vi "HFRR ADV v012 new software.vi"() -> ()   [LabVIEW 2025] (continued)
                n3074 = local read "Ref A Test Date :"() -> (→"TITTLE 4":string)
                n3075 = local read "Temperature before test 3"() -> (w3788:dbl)
                n3076 = local read "Temperature before test 3"() -> (→"Temperature after test 5":dbl)
                n3077 = local read "Temperature after test 3"() -> (→"Temperature after test 4":dbl)
                n3078 = local read "Humidity before test 3"() -> (→"Humidity before test 4":dbl)
                n3079 = local write "Temperature before test 3"(w3788) -> ()
                n3080 = local read "image data"() -> (w3779:T15)
                n3081 = String To Path(string="C:\\LAB-IQ\\im\\Temp_resized.jpg") -> (path=w3780:path)
                "path 2" <- w3780
                n3082 = call <vilib>:"Write JPEG File.vi"("image data"=w3779, "path to JPEG file"=w3780) -> ()  [unwired: 8 in, 2 out]
                "Ref A Test Date :" <- "Ref A Test Date :"
                "Ref B Test Date :" <- "Ref B Test Date :"
                "Ref B Scar Value :" <- "Ref B Scar Value :"
                "Ref A Scar Value :" <- "Ref A Scar Value :"
              }
              frame #1 {
                (unwired) HTML_Report_Image_Alignment."MIDDLE" ("alignment (default)")
                w3816 = u16 0 items=["portrait", "landscape"] ("orientation (portrait)")
                (unwired) HTML_Report_Image_Alignment."ABSMIDDLE" ("alignment (default)")
                (unwired) "TESTED BY : "
                (unwired) "TESTED DATE :"
                (unwired) "SAMPLE ID : "
                (unwired) "SAMPLE DESIGN : "
                w3849 = "\r"
                # "add image"
                n3083 = Wait (ms)(milliseconds to wait=u32 20) -> ()  [unwired: 1 out]
                n3084 = local read "Sample ID  2"() -> (w3842:string)
                n3085 = local read "Wear Scar X"() -> (w3814:dbl)
                "Length ( microns ) 2" <- w3814
                n3086 = local read "Wear Scar Y"() -> (w3813:dbl)
                "Wear Scar Y ( microns ) :" <- w3813
                n3087 = local read "Test Date 2"() -> (w3843:string)
                n3088 = local read "Tested by 2"() -> (w3844:string)
                n3089 = local read "String 46"() -> (w3840:string)
                n3090 = local read "String 48"() -> (w3846:string)
                n3091 = local read "String 47"() -> (w3845:string)
                n3092 = local read "String 49"() -> (w3847:string)
                n3093 = local read "String 10"() -> (w3800:string)
                n3094 = local read "s.NO 2"() -> (w3841:string)
                n3095 = Add(x=w3814, y=w3813) -> (x+y=w3812:dbl)
                n3096 = call <vilib>:"New Report.vi"("report type"=enum16{"Standard Report", "HTML"}."HTML") -> ("report out"=w3820:refnum<class "NI_report.lvclass">, "error out"=w3818:errorcluster)  [unwired: 13 in]
                n3097 = Concatenate Strings(w3849, w3840, w3841, w3849, w3846, w3842, w3849, w3845, w3843, w3849, w3847, w3844, w3849) -> (→"test by 2":string)
                n3098 = Concatenate Strings("C:\\LAB-IQ\\Data\\" ("string"), w3800, ".jpg" ("string")) -> ()  [unwired: 1 out]
                n3099 = Divide(x=w3812, y=2.0) -> (x/y=→"Mean Wear ( microns) :":dbl)
                n3100 = call-dynamic "Set Report Orientation.vi"("report in"=w3820, "orientation (portrait)"=w3816, "error in (no error)"=w3818) -> ("report out"=w3819:refnum<class "NI_report.lvclass">, "error out"=w3817:errorcluster)  [unwired: 11 in]
                n3101 = for {
                  N: 5 -> [_]
                  tunnel: w3819 -> [w3870]
                  tunnel: [w3869] -> w3798
                  tunnel: w3817 -> [w3868]
                  tunnel: [w3867] -> w3797
                  n3102 = call-dynamic "Set Report Tab Width.vi"("report in"=w3870, "error in (no error)"=w3868) -> ("report out"=w3869:refnum<class "NI_report.lvclass">, "error out"=w3867:errorcluster)  [unwired: 12 in]
                }
                n3103 = local read "TITTLE"() -> (w3815:string)
                n3104 = call-dynamic "Set Report Header Text.vi"("report in"=w3798, "center header text"=w3815, "error in (no error)"=w3797) -> ("report out"=w3836:refnum<class "NI_report.lvclass">, "error out"=w3835:errorcluster)  [unwired: 11 in]
                n3105 = for {
                  N: 1 -> [_]
                  tunnel: [w3874] -> w3822
                  tunnel: [w3873] -> w3821
                  tunnel: w3836 -> [w3872]
                  tunnel: w3835 -> [w3871]
                  n3106 = call-dynamic "New Report Line.vi"("report in"=w3872, "error in (no error)"=w3871) -> ("report out"=w3874:refnum<class "NI_report.lvclass">, "error out"=w3873:errorcluster)  [unwired: 12 in]
                }
                n3107 = for {
                  N: 2 -> [_]
                  tunnel: [w3866] -> w3828
                  tunnel: [w3865] -> w3827
                  tunnel: w3822 -> [w3864]
                  tunnel: w3821 -> [w3863]
                  n3108 = call-dynamic "New Report Line.vi"("report in"=w3864, "error in (no error)"=w3863) -> ("report out"=w3866:refnum<class "NI_report.lvclass">, "error out"=w3865:errorcluster)  [unwired: 12 in]
                }
                n3109 = for {
                  N: 25 -> [_]
                  tunnel: w3828 -> [w3862]
                  tunnel: w3827 -> [w3860]
                  tunnel: [w3861] -> w3831
                  tunnel: [w3859] -> w3830
                  n3110 = call-dynamic "Set Report Tab Width.vi"("report in"=w3862, "error in (no error)"=w3860) -> ("report out"=w3861:refnum<class "NI_report.lvclass">, "error out"=w3859:errorcluster)  [unwired: 12 in]
                }
                n3111 = control-ref of="Tab Control 9"() -> (w3826:refnum<vi>)
                n3112 = call-dynamic "Append Control Image to Report.vi"("report in"=w3831, "alignment (default)"=HTML_Report_Image_Alignment."ABSMIDDLE", "ctrl reference"=w3826, "error in (no error)"=w3830) -> ("report out"=w3825:refnum<class "NI_report.lvclass">, "error out"=w3824:errorcluster)  [unwired: 8 in, 2 out]
                n3113 = for {
                  N: 3 -> [_]
                  tunnel: [w3858] -> w3809
                  tunnel: [w3857] -> w3808
                  tunnel: w3825 -> [w3856]
                  tunnel: w3824 -> [w3855]
                  n3114 = call-dynamic "New Report Line.vi"("report in"=w3856, "error in (no error)"=w3855) -> ("report out"=w3858:refnum<class "NI_report.lvclass">, "error out"=w3857:errorcluster)  [unwired: 12 in]
                }
                n3115 = for {
                  N: 100 -> [_]
                  tunnel: w3809 -> [w3854]
                  tunnel: w3808 -> [w3852]
                  tunnel: [w3853] -> w3805
                  tunnel: [w3851] -> w3803
                  n3116 = call-dynamic "Set Report Tab Width.vi"("report in"=w3854, "error in (no error)"=w3852) -> ("report out"=w3853:refnum<class "NI_report.lvclass">, "error out"=w3851:errorcluster)  [unwired: 12 in]
                }
                n3117 = String To Path(string="C:\\LAB-IQ\\im\\Temp_resized.jpg") -> (path=w3795:path)
                n3118 = call-poly <vilib>:"Append Image to Report.vi"("report in"=w3805, "path or URL of image"=w3795, "error in (no error)"=w3803) -> ("report out"=w3804:refnum<class "NI_report.lvclass">, "error out"=w3802:errorcluster)  [unwired: 9 in, 2 out]
                n3119 = call-poly <vilib>:"Open HTML Report in Browser.vi"("report in"=w3804, "error in (no error)"=w3802) -> ("report out"=w3839:refnum<class "NI_report.lvclass">, "error out"=w3838:errorcluster)  [unwired: 11 in, 1 out]
                n3120 = call-dynamic "Dispose Report.vi"("report in"=w3839, "error in (no error)"=w3838) -> ()  [unwired: 13 in, 1 out]
              }
              frame #2 {
              }
              frame #3 {
                n3121 = disable-structure shown="Disabled" {
                  frame Disabled {
                    n3122 = local read "String 10"() -> (w3879:string)
                    n3123 = Concatenate Strings("C:\\LAB-IQ-NXT\\Data\\" ("string"), w3879, ".jpg" ("string")) -> (w3877:string)
                    n3124 = String To Path(string=w3877) -> (path=w3876:path)
                    n3125 = Delete(path (use dialog)=w3876) -> ()  [unwired: 4 in, 3 out]
                  }
                  frame Enabled {
                  }
                }
                n3126 = local write "Print 2"(FALSE ("Print")) -> ()
              }
            }
          }
        }
      }
    }
    n3127 = property on="SetTemp" class="DigNum (strict)"("Disabled"=w1815) -> ()  [unwired: 2 in, 2 out]
    n3128 = Multiply(x=w1805, y=w1807) -> (x*y=w1806:dbl)
    n3129 = local read "MWSD"() -> (w1804:dbl)
    n3130 = Add(x=w1806, y=w1804) -> (x+y=→"WS1.4":dbl)
    n3131 = Wait (ms)(milliseconds to wait=u32 50) -> ()  [unwired: 1 out]
    n3132 = Wait (ms)(milliseconds to wait=u32 50) -> ()  [unwired: 1 out]
    n3133 = local read "Quit"() -> (w1803:bool)
  }
  n3134 = VISA Close(VISA resource name=w52, error in (no error)=w51) -> (error out=w49:errorcluster)
  n3135 = call <vilib>:"Clear Errors.vi"("error in (no error)"=w49) -> ()  [unwired: 5 in, 2 out]
  n3136 = VISA Close(VISA resource name=w37, error in (no error)=w36) -> ()  [unwired: 1 out]
  n3137 = while {
    tunnel: [w4040] -> w46
    shift-right: [w4033] -> _
    shift-left: 0.0 -> [w4036]
    shift-right: [w4032] -> _
    shift-left: 0.0 -> [w4035]
    shift-right: [w4031] -> _
    shift-left: 400.0 ("vc_cmd") -> [w4034]
    stop <- w4040 stop-if-true
    # "PID LOGIC"
    n3138 = local read "RUN"() -> (w4038:bool)
    n3139 = local read "Auto Start Temp"() -> (w4027:bool)
    n3140 = local read "Auto Start Test"() -> (w4037:bool)
    n3141 = local read "START TEMP"() -> (w4029:bool)
    n3142 = And(x=w4027, y=w4037) -> (x .and. y?=w4028:bool)
    n3143 = Or(x=w4038, y=w4028) -> (x .or. y?=w4039:bool)
    n3144 = And(x=w4039, y=w4029) -> (x .and. y?=w4030:bool)
    n3145 = Wait (ms)(milliseconds to wait=u32 20) -> ()  [unwired: 1 out]
    n3146 = case shown="True" w4030 {
      tunnel: [400.0 ("out_vc_cmd") w4060] -> w4031
      tunnel: [w4043 w4062] -> w4032
      tunnel: [w4043 w4061] -> w4033
      tunnel: w4036 -> [_ w4051]
      tunnel: w4035 -> [_ w4050]
      tunnel: w4034 -> [_ w4049]
      frame False {
        w4043 = 0.0 ("error_out")
      }
      frame True {
        n3147 = local read "Set Strk"() -> (w4046:dbl)
        n3148 = local read "LVDT STROKE"() -> (w4044:dbl)
        n3149 = Add(x=w4046, y="Add up Stroke") -> (x+y=w4047:dbl)
        n3150 = formula code="// Zero-Hardcode Explicit Positional-Form PID Engine\n// Inputs: target_stroke, measured_stroke, dt, prev_error, integral_accumulator_in, prev_vc_cmd\n//         kp, ki, kd, max_step_change, max_amplitude, min_amplitude, startup_cmd\n// Outputs: vc_cmd, error_out, out_error, integral_accumulator_out, out_vc_cmd\n\n// 1. Calculate Tracking Error\nfloat current_error = target_stroke - measured_stroke;\nerror_out = current_error;\n\n// 2. Compute Proportional Term\nfloat p_term = kp * current_error;\n\n// 3. Compute Derivative Term\nfloat d_term = 0.0;\nif (dt > 0.0) {\n    d_term = kd * ((current_error - prev_error) / dt);\n}\n\n// 4. Update and Accumulate Integral Term\nfloat current_integral = integral_accumulator_in + (current_error * dt);\nfloat i_term = ki * current_integral;\n\n// 5. Calculate Ideal Target Command\nfloat ideal_command = startup_cmd + p_term + i_term + d_term;\n\n// 6. Anti-Windup Protection (Back-calculation method)\nif (ideal_command > max_amplitude) {\n    float excess = ideal_command - max_amplitude;\n    if (ki > 0.0) {\n        current_integral -= excess / ki;\n    }\n    ideal_command = max_amplitude;\n} else if (ideal_command < min_amplitude) {\n    float excess = ideal_command - min_amplitude;\n    if (ki > 0.0) {\n        current_integral -= excess / ki;\n    }\n    ideal_command = min_amplitude;\n}\n\n// 7. Apply Loop Rate Limiting (Protects voice coil from large voltage steps)\nfloat raw_adjustment = ideal_command - prev_vc_cmd;\n\nif (raw_adjustment > max_step_change) {\n    raw_adjustment = max_step_change;\n} else if (raw_adjustment < -max_step_change) {\n    raw_adjustment = -max_step_change;\n}\n\nfloat next_vc_cmd = prev_vc_cmd + raw_adjustment;\n\n// Final Output Safety Safeguard Clamping\nif (next_vc_cmd > max_amplitude) {\n    next_vc_cmd = max_amplitude;\n} else if (next_vc_cmd < min_amplitude) {\n    next_vc_cmd = min_amplitude;\n}\n\n// 8. Map to Shift Registers for memory persistence\nvc_cmd = next_vc_cmd;\nout_error = current_error;                     \nintegral_accumulator_out = current_integral;  \nout_vc_cmd = next_vc_cmd;"("target_stroke"=w4047, "measured_stroke"=w4044, "dt"="dt", "integral_accumulator_in"=w4050, "prev_error"=w4051, "prev_vc_cmd"=w4049, "kp"="kp", "ki"="ki", "kd"="kd", "max_step_change"="max_step_change", "max_amplitude"="max_amplitude", "min_amplitude"="min_amplitude", "startup_cmd"="startup_cmd") -> ("vc_cmd"=w4066:dbl, "out_error"=w4061:dbl, "integral_accumulator_out"=w4062:dbl, "out_vc_cmd"=w4060:dbl)  [unwired: 1 out]
        "output Vpp" <- w4066
        n3151 = Number To Fractional String(number=w4066, precision (6)=i16 1) -> (F-format string=w4064:string)  [unwired: 2 in]
        n3152 = Concatenate Strings("DAC;" ("string"), w4064) -> (w4048:string)
        n3153 = local write "Command"(w4048) -> ()
        "prev_error" <- w4051
        "integral_accumulator_in" <- w4050
        "prev_vc_cmd" <- w4049
      }
    }
    n3154 = local read "Quit"() -> (w4040:bool)
  }
  n3155 = Or(x=w42, y=w41) -> (x .or. y?=w43:bool)
  n3156 = Or(x=w39, y=w43) -> (x .or. y?=w48:bool)
  n3157 = control-ref of="new picture"() -> ()  [unwired: 1 out]
  n3158 = Or(x=w54, y=w48) -> (x .or. y?=w45:bool)
  n3159 = Or(x=w45, y=w46) -> (x .or. y?=w40:bool)
  n3160 = while {
    tunnel: [w4067] -> w53
    i -> [w4074]
    stop <- w4067 stop-if-true
    n3161 = local read "Quit"() -> (w4067:bool)
    n3162 = Equal To 0?(x=w4074) -> (x = 0?=w4072:bool)
    n3163 = call "Elapsed Time3"("Time Target (s)"=45.0, "Auto Reset"=TRUE) -> ("Time has Elapsed"=w4071:bool)  [unwired: 10 in, 7 out]
    n3164 = Wait (ms)(milliseconds to wait=u32 50) -> ()  [unwired: 1 out]
    n3165 = Or(x=w4071, y=w4072) -> (x .or. y?=w4073:bool)
    n3166 = case shown="True" w4073 {
      frame False {
      }
      frame True {
        n3167 = call <vilib>:"System Exec.vi"("run minimized? (F)"=TRUE, "error in (no error)"="error in (no error)", "command line"="powercfg.exe -change -monitor-timeout-ac 0") -> ("error out"=w4085:errorcluster)  [unwired: 5 in, 3 out]
        n3168 = call <vilib>:"System Exec.vi"("run minimized? (F)"=TRUE, "error in (no error)"=w4085, "command line"="powercfg.exe -change -disk-timeout-ac 0") -> ("error out"=w4084:errorcluster)  [unwired: 5 in, 3 out]
        n3169 = call <vilib>:"System Exec.vi"("run minimized? (F)"=TRUE, "error in (no error)"=w4084, "command line"="powercfg.exe -change -standby-timeout-ac 0") -> ("error out"=w4083:errorcluster)  [unwired: 5 in, 3 out]
        n3170 = call <vilib>:"System Exec.vi"("run minimized? (F)"=TRUE, "error in (no error)"=w4083, "command line"="powercfg.exe -change -hibernate-timeout-ac 0") -> ("error out"=w4082:errorcluster)  [unwired: 5 in, 3 out]
        n3171 = call <vilib>:"Simple Error Handler.vi"("error in (no error)"=w4082) -> ("error out"=w4088:errorcluster)  [unwired: 4 in, 4 out]
        n3172 = call <vilib>:"Clear Errors.vi"("error in (no error)"=w4088) -> ("error out"=→"error out":errorcluster)  [unwired: 5 in, 1 out]
      }
    }
  }
  n3173 = Compound Arithmetic op=OR(w56, w40, w53) -> (w55:bool)
  n3174 = flat-sequence {
    tunnel: w55 -> [_]
    tunnel: [w4090] -> w18
    tunnel: w18 -> [_]
    frame #0 {
      n3175 = call "CLOSE CONNECTION.vi"() -> ("error out"=w4090:errorcluster)  [unwired: 11 in]
    }
    frame #1 {
      n3176 = Quit LabVIEW(quit? (T)=TRUE) -> ()
      n3177 = local write "Quit"(FALSE ("EXIT")) -> ()
    }
  }
  n3178 = property on="Heater Button" class="Bool (strict)"("Visible"=TRUE) -> ()  [unwired: 2 in, 2 out]
  n3179 = disable-structure shown="Disabled" {
    disable-tunnel: _ -> [w4096 _]
    disable-tunnel: _ -> [w4093 _]
    disable-tunnel: _ -> [w4094 _]
    frame Disabled {
      n3180 = disable-structure shown="Disabled" {
        disable-tunnel: [w4103 _] -> w4095
        frame Disabled {
          n3181 = while {
            shift-right: [w4145] -> w4101
            shift-left: errorcluster {"status"=TRUE, "code"=0, "source"="Init"} ("error out") -> [w4110]
            shift-right: [w4144] -> w4100
            shift-left: _ -> [w4111]
            shift-right: [w4143] -> _
            shift-left: "" -> [w4142]
            tunnel: [w4104] -> w4103
            shift-right: ["Set Rh"] -> _
            shift-left: 0.0 ("Set Rh") -> [w4136]
            tunnel: [w4113] -> _
            i -> [w4113]
            stop <- w4104 stop-if-true
            n3182 = flat-sequence {
              tunnel: w4110 -> [w4148]
              tunnel: [w4148] -> w4109
              frame #0 {
                n3183 = Wait (ms)(milliseconds to wait=u32 200) -> ()  [unwired: 1 out]
              }
            }
            n3184 = local read "Com Port 3"() -> (w4112:refnum<visa-resource-name>)
            n3185 = local read "Humidity Str Rec"() -> (w4114:string)
            n3186 = Not Equal?(x="Set Rh", y=w4136) -> (x != y?=w4141:bool)
            n3187 = Number To Decimal String(number="Set Rh") -> (decimal integer string=w4139:string)  [unwired: 1 in]
            n3188 = Not Equal?(x=w4112, y=w4111) -> (x != y?=w4107:bool)
            n3189 = Concatenate Strings("#setPoint00" ("string"), w4139) -> (w4140:string)
            n3190 = case shown="False" w4141 {
              tunnel: w4140 -> [_ w4160]
              frame False {
                n3191 = local read "Humidity"() -> (w4157:bool)
                n3192 = case shown="True" w4157 {
                  frame False {
                    n3193 = local write "Humidity Str Send"("stop" ("Humidity Str Send")) -> ()
                  }
                  frame True {
                    n3194 = local write "Humidity Str Send"("start" ("Humidity Str Send")) -> ()
                  }
                }
              }
              frame True {
                n3195 = local write "Humidity Str Send"(w4160) -> ()
              }
            }
            n3196 = Or(x=w4107) -> (y=w4105:bool, x .or. y?=w4106:bool)
            n3197 = String Subset(string=w4114, offset (0)=7) -> (substring=w4129:string)  [unwired: 1 in]
            n3198 = Match Pattern(string=w4114, regular expression="?") -> (offset past match=w4132:i32)  [unwired: 1 in, 3 out]
            n3199 = Match Pattern(string=w4114, regular expression="v") -> (offset past match=w4135:i32)  [unwired: 1 in, 3 out]
            n3200 = case shown="True" w4106 {
              tunnel: w4109 -> [w4146 _]
              tunnel: [w4146 errorcluster {"status"=TRUE, "code"=0, "source"="Init"} ("error out")] -> w4108
              frame False {
              }
              frame True {
              }
            }
            n3201 = Equal?(x=w4132, y=-1) -> (x = y?=w4116:bool)
            n3202 = Match Pattern(string=w4129, regular expression="g") -> (after substring=w4130:string, offset past match=w4121:i32)  [unwired: 1 in, 2 out]
            n3203 = Match Pattern(string=w4129, regular expression="y") -> (after substring=w4128:string, offset past match=w4122:i32)  [unwired: 1 in, 2 out]
            n3204 = Greater?(x=w4122, y=w4121) -> (0:w4127:bool)
            n3205 = Greater Or Equal To 0?(x=w4122) -> (x >= 0?=w4119:bool)
            n3206 = Greater Or Equal To 0?(x=w4121) -> (x >= 0?=w4120:bool)
            n3207 = Or(x=w4119, y=w4120) -> (x .or. y?=w4118:bool)
            n3208 = Greater Or Equal To 0?(x=w4135) -> (x >= 0?=w4117:bool)
            n3209 = Select(t=w4128, s=w4127, f=w4130) -> (s? t:f=w4123:string)
            n3210 = case shown="Error" w4108 {
              selector: w4108 -> [w4173 w4219]
              tunnel: [w4171 w4212] -> w4145
              tunnel: w4111 -> [w4174 w4218]
              tunnel: [w4172 w4221] -> w4144
              tunnel: w4142 -> [w4161 w4220]
              tunnel: [w4168 w4220] -> w4143
              frame No Error {
                n3211 = call "Elapsed Time7"() -> ("Time has Elapsed"=w4167:bool)  [unwired: 12 in, 7 out]
                n3212 = Not Equal?(x="Humidity Str Send", y=w4161) -> (x != y?=w4163:bool)
                n3213 = Or(x=w4163, y=w4167) -> (x .or. y?=w4166:bool)
                n3214 = Select(t="Humidity Str Send", s=w4163, f="vals" ("regular expression")) -> (s? t:f=w4162:string)
                n3215 = Or(x=w4166, y="Send") -> (x .or. y?=w4170:bool)
                n3216 = case shown="True" w4170 {
                  tunnel: [w4177 w4182] -> w4171
                  tunnel: w4174 -> [w4176 w4190]
                  tunnel: w4173 -> [w4177 w4189]
                  tunnel: [w4176 w4183] -> w4172
                  tunnel: w4162 -> [_ w4188]
                  tunnel: [w4175 w4179] -> w4168
                  tunnel: "Humidity Str Send" -> [_ w4180]
                  tunnel: w4163 -> [_ w4181]
                  tunnel: w4161 -> [w4175 w4178]
                  frame False {
                  }
                  frame True {
                    n3217 = flat-sequence {
                      tunnel: w4190 -> [w4198]
                      tunnel: w4189 -> [w4197]
                      tunnel: w4188 -> [w4194]
                      tunnel: [w4196] -> w4187
                      tunnel: [w4195] -> w4186
                      tunnel: w4187 -> [w4201]
                      tunnel: w4186 -> [w4200]
                      tunnel: [w4201] -> w4185
                      tunnel: [w4200] -> w4184
                      tunnel: w4185 -> [w4208]
                      tunnel: w4184 -> [w4207]
                      tunnel: [w4206] -> w4183
                      tunnel: [w4205] -> w4182
                      frame #0 {
                        n3218 = local write "Ser Led"(TRUE ("Boolean 4")) -> ()
                        n3219 = Concatenate Strings(w4194, "\r") -> (w4193:string)
                        n3220 = VISA Write(VISA resource name=w4198, write buffer=w4193, error in (no error)=w4197) -> (VISA resource name out=w4196:refnum<visa-resource-name>, error out=w4195:errorcluster)  [unwired: 1 out]
                      }
                      frame #1 {
                        n3221 = Wait (ms)(milliseconds to wait="wait") -> ()  [unwired: 1 out]
                      }
                      frame #2 {
                        w4203 = FALSE ("Send")
                        n3222 = property class="Instr"(reference=w4208, error in=w4207) -> (reference out=w4209:refnum<visa-resource-name>, error out=w4210:errorcluster, "Serial Settings:Number of Bytes at Serial Port"=w4202:u32)
                        n3223 = local write "Send"(w4203) -> ()
                        n3224 = local write "Ser Led"(w4203) -> ()
                        n3225 = VISA Read(VISA resource name=w4209, byte count=w4202, error in (no error)=w4210) -> (VISA resource name out=w4206:refnum<visa-resource-name>, read buffer=→"Humidity Str Rec":string, error out=w4205:errorcluster)  [unwired: 1 out]
                      }
                    }
                    n3226 = Select(t=w4180, s=w4181, f=w4178) -> (s? t:f=w4179:string)
                  }
                }
              }
              frame Error {
                w4226 = u16 0 items=["None"=0, "XON/XOFF"=1, "RTS/CTS"=2, "DTR/DSR"=4] ("flow control")
                w4222 = u16 0 items=["None", "Odd", "Even", "Mark", "Space"] ("parity")
                w4225 = u16 10 items=["1.0"=10, "1.5"=15, "2.0"=20] ("stop bits")
                n3227 = VISA Close(VISA resource name=w4218, error in (no error)=w4219) -> (error out=w4217:errorcluster)
                n3228 = local write "humid"("" ("humid")) -> ()
                n3229 = local write "Humidity Str Rec"("" ("Humidity Str Rec")) -> ()
                n3230 = call <vilib>:"Clear Errors.vi"("error in (no error)"=w4217) -> ("error out"=w4216:errorcluster)  [unwired: 5 in, 1 out]
                n3231 = local read "Com Port 3"() -> (w4215:refnum<visa-resource-name>)
                n3232 = call-poly "VISA Configure Serial Port"("VISA resource name"=w4215, "timeout (10sec)"=u32 1000, "termination char\n(0xA = '\\n' = LF)"=u8 10 ("termination char\n(0xA = '\\n' = LF)"), "Enable Termination\nChar (T)"=FALSE ("Enable Termination Char (T)"), "data bits (8)"=u16 8 ("data bits"), "parity (0:none)"=w4222, "error in (no error)"=w4216, "stop bits (10: 1 bit)"=w4225, "flow control (0:none)"=w4226) -> ("VISA resource name out"=w4221:refnum<visa-resource-name>, "baud rate (9600)"=w4213:u32, "error out"=w4212:errorcluster)  [unwired: 4 in]
              }
            }
            n3233 = Compound Arithmetic op=AND(w4117, w4116, w4118) -> (w4115:bool)
            n3234 = case shown="True" w4115 {
              tunnel: w4114 -> [_ _]
              tunnel: w4123 -> [_ w4153]
              frame False {
              }
              frame True {
                w4151 = " " ("regular expression")
                n3235 = Match Pattern(string=w4153, regular expression=" ") -> (after substring=w4155:string)  [unwired: 1 in, 3 out]
                n3236 = Match Pattern(string=w4155, regular expression=w4151) -> (before substring=→"humid":string, after substring=w4152:string)  [unwired: 1 in, 2 out]
                n3237 = Match Pattern(string=w4152, regular expression=w4151) -> (before substring=→"temp_@Rh sensor":string)  [unwired: 1 in, 3 out]
              }
            }
            n3238 = local read "Quit"() -> (w4104:bool)
          }
          n3239 = VISA Close(VISA resource name=w4100, error in (no error)=w4101) -> (error out=w4097:errorcluster)
          n3240 = call <vilib>:"Clear Errors.vi"("error in (no error)"=w4097) -> ()  [unwired: 5 in, 2 out]
        }
        frame Enabled {
        }
      }
    }
    frame Enabled {
    }
  }
  n3241 = while {
    tunnel: [w4233] -> _
    i -> [w4233]
    stop <- w4229 stop-if-true
    # "Langauage selection"
    n3242 = Equal?(x="Lan flag", y=22.0) -> ()  [unwired: 1 out]
    n3243 = disable-structure shown="Disabled" {
      frame Disabled {
        n3244 = stacked-sequence {
          frame #0 {
            n3245 = case shown="\"Russian\"" "Language Selection" {
              tunnel: [0 1] -> w4235
              frame "English", Default {
              }
              frame "Russian" {
              }
            }
            n3246 = for {
              N: 130 -> [_]
              tunnel: "Table" -> [w4244]
              tunnel: w4235 -> [w4243]
              i -> [w4242]
              n3247 = Index Array(array=w4244, index (row)=w4242, index (col)=w4243) -> (element=w4241:string)
              n3248 = case shown="123" w4242 {
                tunnel: w4241 -> [w4245 w4246 _ w4247 w4248 w4249 w4250 w4251 w4252 w4253 w4254 w4255 w4256 w4257 w4258 w4259 w4260 w4261 w4262 w4263 w4264 w4265 w4266 w4267 w4268 w4269 w4270 w4271 w4272 _ _ w4273 w4274 w4275 w4276 w4277 w4278 w4287 w4294 w4301 w4308 w4312 w4315 w4318 w4320 w4322 w4323 w4324 w4325 w4326 w4327 w4328 w4329 w4330 w4331 w4332 w4333 w4334 w4335 w4336 w4337 w4338 w4339 w4340 w4341 w4342 w4343 w4344 w4345 w4346 w4347 w4348 w4349 w4350 w4351 w4352 w4353 w4354 w4355 w4356 w4357 w4358 w4359 w4360 w4361 w4362 w4363 w4364 w4365 w4366 w4367 w4368 w4369 w4370 w4371 w4372 w4373 w4374 w4375 w4376 w4377 w4378 w4379 w4380 w4381 _ w4382 w4383 w4384 w4385 w4386 w4387 w4388 w4389 w4390 w4391 w4392 w4393 w4394 _ w4395 w4396 w4397 w4398 w4399 w4400 _]
                frame 0 {
                  n3249 = local write "S"(w4245) -> ()
                }
                frame 1 {
                  n3250 = local write "S 2"(w4246) -> ()
                }
                frame 2 {
                }
                frame 3 {
                  n3251 = local write "S 4"(w4247) -> ()
                }
                frame 4 {
                  n3252 = property on="FILE" class="Str"("Caption.Text"=w4248) -> ()  [unwired: 2 in, 2 out]
                }
                frame 5 {
                  n3253 = property on="Fuel Discription :" class="Str"("Caption.Text"=w4249) -> ()  [unwired: 2 in, 2 out]
                }
                frame 6 {
                  n3254 = property on="Remarks :" class="Str"("Caption.Text"=w4250) -> ()  [unwired: 2 in, 2 out]
                }
                frame 7 {
                  n3255 = property on="Save & Continue" class="Bool (strict)"("Boolean Text.Text"=w4251) -> ()  [unwired: 2 in, 2 out]
                }
                frame 8 {
                }
                frame 9 {
                  n3256 = property on="Set Hz" class="DigNum (strict)"("Caption.Text"=w4253) -> ()  [unwired: 2 in, 2 out]
                }
                frame 10 {
                  "String 3" <- w4254
                }
                frame 11 {
                  n3257 = property on="NORMAL LOAD" class="DigNum (strict)"("Caption.Text"=w4255) -> ()  [unwired: 2 in, 2 out]
                }
                frame 12 {
                  "String 5" <- w4256
                }
                frame 13 {
                  n3258 = property on="Set Temp" class="DigNum (strict)"("Caption.Text"=w4257) -> ()  [unwired: 2 in, 2 out]
                }
                frame 14 {
                  n3259 = local write "S 15"(w4258) -> ()
                }
                frame 15 {
                  n3260 = property on="Set Rh" class="DigNum (strict)"("Caption.Text"=w4259) -> ()  [unwired: 2 in, 2 out]
                }
                frame 16 {
                  "String 13" <- w4260
                  "String 26" <- w4260
                }
                frame 17 {
                  n3261 = local write "S 18"(w4261) -> ()
                }
                frame 18 {
                  "String 17" <- w4262
                }
                frame 19 {
                  n3262 = property on="test time" class="DigNum (strict)"("Caption.Text"=w4263) -> ()  [unwired: 2 in, 2 out]
                }
                frame 20 {
                  "String 18" <- w4264
                  "String 22" <- w4264
                }
                frame 21 {
                  n3263 = property on="Elapsed time" class="DigNum (strict)"("Caption.Text"=w4265) -> ()  [unwired: 2 in, 2 out]
                }
                frame 22 {
                  n3264 = property on="Samplingtime 2" class="DigNum (strict)"("Caption.Text"=w4266) -> ()  [unwired: 2 in, 2 out]
                }
                frame 23 {
                  "String 21" <- w4267
                }
                frame 24 {
                  n3265 = property on="Countdown" class="DigNum (strict)"("Caption.Text"=w4268) -> ()  [unwired: 2 in, 2 out]
                }
                frame 25 {
                  n3266 = property on="Countdown 2" class="DigNum (strict)"("Caption.Text"=w4269) -> ()  [unwired: 2 in, 2 out]
                }
                frame 26 {
                  n3267 = property on="Engage" class="Bool (strict)"("Boolean Text.Text"=w4270) -> ()  [unwired: 2 in, 2 out]
                }
                frame 27 {
                  n3268 = property on="Boolean  4" class="Bool (strict)"("Boolean Text.Text"=w4271) -> ()  [unwired: 2 in, 2 out]
                }
                frame 28 {
                  n3269 = property on="Test \nStatus" class="Bool (strict)"("Boolean Text.Text"=w4272) -> ()  [unwired: 2 in, 2 out]
                }
                frame 29 {
                }
                frame 30 {
                }
                frame 31 {
                }
                frame 32 {
                  n3270 = property on="RSTCOF" class="Bool"("Boolean Text.Text"=w4274) -> ()  [unwired: 2 in, 2 out]
                  n3271 = property on="RST FF" class="Bool"("Boolean Text.Text"=w4274) -> ()  [unwired: 2 in, 2 out]
                  n3272 = property on="RST TEMP" class="Bool"("Boolean Text.Text"=w4274) -> ()  [unwired: 2 in, 2 out]
                  n3273 = property on="RSTV1 3" class="Bool"("Boolean Text.Text"=w4274) -> ()  [unwired: 2 in, 2 out]
                  n3274 = property on="rstv2" class="Bool"("Boolean Text.Text"=w4274) -> ()  [unwired: 2 in, 2 out]
                  n3275 = property on="RSTV1 2" class="Bool"("Boolean Text.Text"=w4274) -> ()  [unwired: 2 in, 2 out]
                  n3276 = property on="RST CP" class="Bool"("Boolean Text.Text"=w4274) -> ()  [unwired: 2 in, 2 out]
                }
                frame 33 {
                  "S 61" <- w4275
                }
                frame 34 {
                  "String 23" <- w4276
                }
                frame 35 {
                  n3277 = property on="Rh Before" class="DigNum (strict)"("Caption.Text"=w4277) -> ()  [unwired: 2 in, 2 out]
                }
                frame 36 {
                  n3278 = Match Pattern(string=w4278, regular expression=",") -> (before substring=→"bs":string, after substring=→"as":string)  [unwired: 1 in, 2 out]
                  n3279 = property on="Rh After" class="DigNum (strict)"("Caption.Text"=w4278) -> ()  [unwired: 2 in, 2 out]
                }
                frame 37 {
                  n3280 = Match Pattern(string=w4287, regular expression=",") -> (before substring=w4286:string, after substring=w4285:string)  [unwired: 1 in, 2 out]
                  "bs" <- w4286
                  "as" <- w4285
                  n3281 = Concatenate Strings(w4286, w4285) -> (w4282:string)
                  n3282 = property on="Humidity before test 2" class="DigNum (strict)"("Caption.Text"=w4282) -> ()  [unwired: 2 in, 2 out]
                  n3283 = property on="Humidity before test" class="DigNum (strict)"("Caption.Text"=w4282) -> ()  [unwired: 2 in, 2 out]
                  n3284 = Concatenate Strings(w4282, "=" ("string")) -> (w4283:string)
                  n3285 = local write "S 38"(w4283) -> ()
                }
                frame 38 {
                  n3286 = Match Pattern(string=w4294, regular expression=",") -> (before substring=w4293:string, after substring=w4292:string)  [unwired: 1 in, 2 out]
                  "bs" <- w4293
                  "as" <- w4292
                  n3287 = Concatenate Strings(w4293, w4292) -> (w4289:string)
                  n3288 = property on="Humidity after test 2" class="DigNum (strict)"("Caption.Text"=w4289) -> ()  [unwired: 2 in, 2 out]
                  n3289 = Concatenate Strings(w4289, "=" ("string")) -> (w4291:string)
                  n3290 = property on="Humidity after test" class="DigNum (strict)"("Caption.Text"=w4289) -> ()  [unwired: 2 in, 2 out]
                  n3291 = local write "S 39"(w4291) -> ()
                }
                frame 39 {
                  n3292 = Match Pattern(string=w4301, regular expression=",") -> (before substring=w4300:string, after substring=w4299:string)  [unwired: 1 in, 2 out]
                  "bs" <- w4300
                  "as" <- w4299
                  n3293 = Concatenate Strings(w4300, w4299) -> (w4296:string)
                  n3294 = property on="Temperature before test 2" class="DigNum (strict)"("Caption.Text"=w4296) -> ()  [unwired: 2 in, 2 out]
                  n3295 = property on="Temperature before test" class="DigNum (strict)"("Caption.Text"=w4296) -> ()  [unwired: 2 in, 2 out]
                  n3296 = Concatenate Strings(w4296, "=" ("string")) -> (→"String 34":string)
                }
                frame 40 {
                  n3297 = Match Pattern(string=w4308, regular expression=",") -> (before substring=w4307:string, after substring=w4306:string)  [unwired: 1 in, 2 out]
                  "bs" <- w4307
                  "as" <- w4306
                  n3298 = Concatenate Strings(w4307, w4306) -> (w4303:string)
                  n3299 = property on="Temperature after test 2" class="DigNum (strict)"("Caption.Text"=w4303) -> ()  [unwired: 2 in, 2 out]
                  n3300 = Concatenate Strings(w4303, "=" ("string")) -> (→"String 35":string)
                  n3301 = property on="Temperature after test" class="DigNum (strict)"("Caption.Text"=w4303) -> ()  [unwired: 2 in, 2 out]
                }
                frame 41 {
                  n3302 = property on="AVP" class="DigNum (strict)"("Caption.Text"=w4312) -> ()  [unwired: 2 in, 2 out]
                  n3303 = property on="AVP 2" class="DigNum (strict)"("Caption.Text"=w4312) -> ()  [unwired: 2 in, 2 out]
                  n3304 = Concatenate Strings(w4312, "=" ("string")) -> (→"String 36":string)
                }
                frame 42 {
                  n3305 = property on="MWSD" class="DigNum (strict)"("Caption.Text"=w4315) -> ()  [unwired: 2 in, 2 out]
                  n3306 = property on="MWSD 2" class="DigNum (strict)"("Caption.Text"=w4315) -> ()  [unwired: 2 in, 2 out]
                  n3307 = Concatenate Strings(w4315, "=" ("string")) -> (→"String 37":string)
                }
                frame 43 {
                  n3308 = property on="HCF 2" class="DigNum (strict)"("Caption.Text"=w4318) -> ()  [unwired: 2 in, 2 out]
                  n3309 = property on="HCF" class="DigNum (strict)"("Caption.Text"=w4318) -> ()  [unwired: 2 in, 2 out]
                  n3310 = Concatenate Strings(w4318, "=" ("string")) -> (→"String 38":string)
                }
                frame 44 {
                  n3311 = Concatenate Strings(w4320, "=" ("string")) -> (→"String 39":string)
                  n3312 = property on="WS1.4 2" class="DigNum (strict)"("Caption.Text"=w4320) -> ()  [unwired: 2 in, 2 out]
                  n3313 = property on="WS1.4" class="DigNum (strict)"("Caption.Text"=w4320) -> ()  [unwired: 2 in, 2 out]
                }
                frame 45 {
                  n3314 = property on="Save Results" class="Bool (strict)"("Boolean Text.Text"=w4322) -> ()  [unwired: 2 in, 2 out]
                }
                frame 46 {
                  n3315 = local write "S 47"(w4323) -> ()
                }
                frame 47 {
                  n3316 = local write "S 48"(w4324) -> ()
                }
                frame 48 {
                  n3317 = local write "S 49"(w4325) -> ()
                }
                frame 49 {
                  n3318 = local write "S 50"(w4326) -> ()
                }
                frame 50 {
                  n3319 = local write "S 51"(w4327) -> ()
                }
                frame 51 {
                  n3320 = local write "S 52"(w4328) -> ()
                }
                frame 52 {
                  n3321 = local write "S 53"(w4329) -> ()
                }
                frame 53 {
                  n3322 = local write "S 54"(w4330) -> ()
                }
                frame 54 {
                  n3323 = local write "S 55"(w4331) -> ()
                }
                frame 55 {
                  n3324 = local write "S 56"(w4332) -> ()
                }
                frame 56 {
                  n3325 = local write "S 57"(w4333) -> ()
                }
                frame 57 {
                  n3326 = local write "S 58"(w4334) -> ()
                }
                frame 58 {
                  n3327 = local write "S 59"(w4335) -> ()
                }
                frame 59 {
                  n3328 = local write "S 60"(w4336) -> ()
                }
                frame 60 {
                  n3329 = local write "S 62"(w4337) -> ()
                }
                frame 61 {
                  n3330 = local write "S 63"(w4338) -> ()
                }
                frame 62 {
                  n3331 = local write "S 64"(w4339) -> ()
                }
                frame 63 {
                  n3332 = local write "S 65"(w4340) -> ()
                }
                frame 64 {
                  n3333 = local write "S 66"(w4341) -> ()
                }
                frame 65 {
                  n3334 = local write "S 67"(w4342) -> ()
                }
                frame 66 {
                  n3335 = local write "S 68"(w4343) -> ()
                }
                frame 67 {
                  n3336 = local write "S 69"(w4344) -> ()
                }
                frame 68 {
                  n3337 = local write "S 70"(w4345) -> ()
                }
                frame 69 {
                  n3338 = local write "S 71"(w4346) -> ()
                }
                frame 70 {
                  n3339 = local write "S 72"(w4347) -> ()
                }
                frame 71 {
                  n3340 = local write "S 73"(w4348) -> ()
                }
                frame 72 {
                  n3341 = local write "S 74"(w4349) -> ()
                }
                frame 73 {
                  n3342 = local write "S 75"(w4350) -> ()
                }
                frame 74 {
                  n3343 = local write "S 76"(w4351) -> ()
                }
                frame 75 {
                  n3344 = local write "S 77"(w4352) -> ()
                }
                frame 76 {
                  n3345 = local write "S 78"(w4353) -> ()
                }
                frame 77 {
                  n3346 = local write "S 79"(w4354) -> ()
                }
                frame 79 {
                  n3347 = property on="Sample Temperature ( °C )" class="XYGraph (strict)"("Y Scale.Name Label.Text"=w4355) -> ()  [unwired: 2 in, 2 out]
                }
                frame 80 {
                  n3348 = local write "S 81"(w4356) -> ()
                  n3349 = property on="Humidity ( %RH )" class="XYGraph (strict)"("Y Scale.Name Label.Text"=w4356) -> ()  [unwired: 2 in, 2 out]
                }
                frame 78 {
                  n3350 = property on="Air Temperature  ( °C )" class="XYGraph (strict)"("X Scale.Name Label.Text"=w4357) -> ()  [unwired: 2 in, 2 out]
                  n3351 = property on="Humidity ( %RH )" class="XYGraph (strict)"("X Scale.Name Label.Text"=w4357) -> ()  [unwired: 2 in, 2 out]
                  n3352 = property on="Sample Temperature ( °C )" class="XYGraph (strict)"("X Scale.Name Label.Text"=w4357) -> ()  [unwired: 2 in, 2 out]
                  n3353 = property on="Coefficient Of Friction" class="XYGraph (strict)"("X Scale.Name Label.Text"=w4357) -> ()  [unwired: 2 in, 2 out]
                }
                frame 81 {
                  n3354 = property on="Air Temperature  ( °C )" class="XYGraph (strict)"("Y Scale.Name Label.Text"=w4358) -> ()  [unwired: 2 in, 2 out]
                }
                frame 82 {
                  n3355 = local write "S 84"(w4359) -> ()
                }
                frame 83 {
                  n3356 = local write "S 85"(w4360) -> ()
                }
                frame 84 {
                  n3357 = local write "S 86"(w4361) -> ()
                }
                frame 85 {
                  n3358 = local write "S 87"(w4362) -> ()
                }
                frame 86 {
                  n3359 = local write "S 88"(w4363) -> ()
                }
                frame 87 {
                }
                frame 88 {
                  n3360 = local write "S 90"(w4365) -> ()
                }
                frame 89 {
                  n3361 = local write "S 91"(w4366) -> ()
                }
                frame 90 {
                  n3362 = local write "S 92"(w4367) -> ()
                }
                frame 91 {
                  n3363 = local write "S 93"(w4368) -> ()
                }
                frame 92 {
                  n3364 = local write "S 94"(w4369) -> ()
                }
                frame 93 {
                  n3365 = local write "S 95"(w4370) -> ()
                }
                frame 94 {
                  n3366 = local write "S 96"(w4371) -> ()
                }
                frame 95 {
                  n3367 = local write "S 97"(w4372) -> ()
                }
                frame 96 {
                  n3368 = local write "S 98"(w4373) -> ()
                }
                frame 97 {
                  n3369 = local write "S 99"(w4374) -> ()
                }
                frame 98 {
                  n3370 = local write "S 100"(w4375) -> ()
                }
                frame 99 {
                  n3371 = local write "S 101"(w4376) -> ()
                }
                frame 100 {
                  n3372 = local write "S 102"(w4377) -> ()
                }
                frame 101 {
                  n3373 = local write "S 103"(w4378) -> ()
                }
                frame 102 {
                  n3374 = local write "S 104"(w4379) -> ()
                }
                frame 103 {
                  n3375 = local write "S 105"(w4380) -> ()
                }
                frame 104 {
                  n3376 = local write "S 106"(w4381) -> ()
                }
                frame 105 {
                }
                frame 106 {
                  n3377 = property on="OK Button 17" class="Bool (strict)"("Boolean Text.Text"=w4382) -> ()  [unwired: 2 in, 2 out]
                }
                frame 107 {
                  n3378 = property on="OK Button 16" class="Bool (strict)"("Boolean Text.Text"=w4383) -> ()  [unwired: 2 in, 2 out]
                }
                frame 108 {
                  n3379 = property on="TITTLE" class="Str"("Caption.Text"=w4384) -> ()  [unwired: 2 in, 2 out]
                }
                frame 109 {
                  "String 30" <- w4385
                }
                frame 110 {
                  n3380 = property on="Test Date" class="Str"("Caption.Text"=w4386) -> ()  [unwired: 2 in, 2 out]
                  "String 31" <- w4386
                }
                frame 111 {
                  n3381 = property on="Sample ID" class="Str"("Caption.Text"=w4387) -> ()  [unwired: 2 in, 2 out]
                  "String 32" <- w4387
                }
                frame 112 {
                  n3382 = property on="Tested by" class="Str"("Caption.Text"=w4388) -> ()  [unwired: 2 in, 2 out]
                  "String 33" <- w4388
                }
                frame 113 {
                  n3383 = property on="System Configured Printers 2" class="Arr (strict)"("Caption.Text"=w4389) -> ()  [unwired: 2 in, 2 out]
                }
                frame 114 {
                  n3384 = property on="Selected Printer" class="Str"("Caption.Text"=w4390) -> ()  [unwired: 2 in, 2 out]
                }
                frame 115 {
                  n3385 = property on="Select Printer 3" class="DigNum (strict)"("Caption.Text"=w4391) -> ()  [unwired: 2 in, 2 out]
                }
                frame 116 {
                  n3386 = property on="Print" class="Bool (strict)"("Boolean Text.Text"=w4392) -> ()  [unwired: 2 in, 2 out]
                }
                frame 117 {
                  "String 41" <- w4393
                }
                frame 118 {
                  n3387 = property on="tested by" class="Str"("Caption.Text"=w4394) -> ()  [unwired: 2 in, 2 out]
                }
                frame 119 {
                }
                frame 120 {
                  n3388 = property on="Export" class="Bool (strict)"("Boolean Text.Text"=w4395) -> ()  [unwired: 2 in, 2 out]
                }
                frame 121 {
                  n3389 = property on="TEMP INTERCEPT:" class="DigNum (strict)"("Caption.Text"=w4396) -> ()  [unwired: 2 in, 2 out]
                }
                frame 122 {
                  n3390 = property on="AIR TEMP INTERCEPT:" class="DigNum (strict)"("Caption.Text"=w4397) -> ()  [unwired: 2 in, 2 out]
                }
                frame 123 {
                  n3391 = property on="Select File Type" class="Enum (strict)"("Caption.Text"=w4398) -> ()  [unwired: 2 in, 2 out]
                }
                frame 124 {
                  n3392 = property on="s.NO" class="Str"("Caption.Text"=w4399) -> ()  [unwired: 2 in, 2 out]
                  "String 45" <- w4399
                }
                frame 125 {
                  n3393 = property on="trip1 8" class="Bool (strict)"("Boolean Text.Text"=w4400) -> ()  [unwired: 2 in, 2 out]
                }
                frame 126, Default {
                }
              }
            }
          }
          frame #1 {
            w4408 = TRUE ("Visible")
            n3394 = local read "S 91"() -> (w4425:string)
            n3395 = local read "S 90"() -> (w4424:string)
            n3396 = local read "S 88"() -> (w4423:string)
            n3397 = property on="File Path" class="Path"("Caption.Text"=w4424) -> ()  [unwired: 2 in, 2 out]
            n3398 = property on="SrvM CP" class="Bool (strict)"("Boolean Text.Text"=w4423) -> ()  [unwired: 2 in, 2 out]
            n3399 = local read "S 71"() -> (w4418:string)
            n3400 = local read "S 86"() -> (w4420:string)
            n3401 = local read "S 85"() -> (w4421:string)
            n3402 = local read "S 87"() -> (w4419:string)
            n3403 = local read "S 84"() -> (w4422:string)
            n3404 = local read "S 103"() -> (w4407:string)
            n3405 = local read "S 104"() -> (w4406:string)
            n3406 = property on="ENTER THE NEW PASSWORD" class="Str"("Caption.Text"=w4419) -> ()  [unwired: 2 in, 2 out]
            n3407 = property on="Password" class="Str"("Caption.Text"=w4421) -> ()  [unwired: 2 in, 2 out]
            n3408 = property on="ENTER CURRENT PASSWORD" class="Str"("Caption.Text"=w4420) -> ()  [unwired: 2 in, 2 out]
            n3409 = property on="EDIT" class="Bool (strict)"("Boolean Text.Text"=w4418) -> ()  [unwired: 2 in, 2 out]
            n3410 = property on="SAVE" class="Bool (strict)"("Boolean Text.Text"=w4422) -> ()  [unwired: 2 in, 2 out]
            n3411 = Build Array(w4407, w4406) -> (w4405:string[])
            n3412 = property on="Heater Button" class="Bool (strict)"("Strings [4]"=w4405) -> ()  [unwired: 2 in, 2 out]
            n3413 = property on="CH-HUMIDITY WET" class="DigNum (strict)"("Caption.Size to Text?"=w4408) -> ()  [unwired: 2 in, 2 out]
            n3414 = property on="CH-HUMIDITY DRY" class="DigNum (strict)"("Caption.Size to Text?"=w4408) -> ()  [unwired: 2 in, 2 out]
            n3415 = property on="CH-POWER -" class="DigNum (strict)"("Caption.Size to Text?"=w4408) -> ()  [unwired: 2 in, 2 out]
            n3416 = property on="CH-HEATER" class="DigNum (strict)"("Caption.Size to Text?"=w4408) -> ()  [unwired: 2 in, 2 out]
            n3417 = property on="CH-POWER +" class="DigNum (strict)"("Caption.Size to Text?"=w4408) -> ()  [unwired: 2 in, 2 out]
            n3418 = local read "S 92"() -> (w4417:string)
            n3419 = local read "S 93"() -> (w4416:string)
            n3420 = local read "S 105"() -> (w4403:string)
            n3421 = local read "S 106"() -> (w4402:string)
            n3422 = Build Array(w4417, w4416) -> ()  [unwired: 1 out]
            n3423 = Build Array(w4403, w4402) -> (w4404:string[])
            n3424 = local read "S 95"() -> (w4414:string)
            n3425 = local read "S 94"() -> (w4415:string)
            n3426 = local read "bs"() -> (w4430:string)
            n3427 = local read "as"() -> (w4431:string)
            n3428 = property on="Humidity" class="Bool (strict)"("Strings [4]"=w4404) -> ()  [unwired: 2 in, 2 out]
            n3429 = Concatenate Strings(w4430, "\r", w4431) -> ()  [unwired: 1 out]
            n3430 = property on="STROKE GAIN :" class="DigNum (strict)"("Caption.Text"=w4414) -> ()  [unwired: 2 in, 2 out]
            n3431 = property on="DISPLACEMENT :" class="DigNum (strict)"("Caption.Text"=w4415) -> ()  [unwired: 2 in, 2 out]
            n3432 = property on="Rh After" class="DigNum (strict)"("Caption.Size to Text?"=TRUE ("Caption.Size to Text")) -> ()  [unwired: 2 in, 2 out]
            n3433 = local read "S 48"() -> (w4454:string)
            n3434 = local read "S 50"() -> (w4452:string)
            n3435 = local read "S 51"() -> (w4451:string)
            n3436 = local read "S 49"() -> (w4453:string)
            n3437 = local read "S 52"() -> (w4450:string)
            n3438 = local read "as"() -> (w4435:string)
            n3439 = local read "bs"() -> (w4436:string)
            n3440 = local read "S 56"() -> (w4449:string)
            n3441 = local read "S 57"() -> (w4448:string)
            n3442 = local read "S 58"() -> (w4447:string)
            n3443 = local read "S 59"() -> (w4446:string)
            n3444 = property on="OPEN" class="Bool (strict)"("Boolean Text.Text"=w4450) -> ()  [unwired: 2 in, 2 out]
            n3445 = property on="OPEN 1" class="Bool (strict)"("Boolean Text.Text"=w4454) -> ()  [unwired: 2 in, 2 out]
            n3446 = property on="OPEN 2" class="Bool (strict)"("Boolean Text.Text"=w4453) -> ()  [unwired: 2 in, 2 out]
            n3447 = property on="OPEN 3" class="Bool (strict)"("Boolean Text.Text"=w4452) -> ()  [unwired: 2 in, 2 out]
            n3448 = property on="OPEN 4" class="Bool (strict)"("Boolean Text.Text"=w4451) -> ()  [unwired: 2 in, 2 out]
            n3449 = Concatenate Strings(w4436, "\r", w4435) -> ()  [unwired: 1 out]
            n3450 = local read "S 102"() -> (w4409:string)
            n3451 = property on="КОФ1" class="DigNum (strict)"("Caption.Text"=w4449) -> ()  [unwired: 2 in, 2 out]
            n3452 = local read "S 98"() -> (w4413:string)
            n3453 = local read "S 99"() -> (w4412:string)
            n3454 = local read "S 100"() -> (w4411:string)
            n3455 = local read "S 101"() -> (w4410:string)
            n3456 = property on="КОФ2" class="DigNum (strict)"("Caption.Text"=w4448) -> ()  [unwired: 2 in, 2 out]
            n3457 = property on="КОФ3" class="DigNum (strict)"("Caption.Text"=w4447) -> ()  [unwired: 2 in, 2 out]
            n3458 = property on="КОФ4" class="DigNum (strict)"("Caption.Text"=w4446) -> ()  [unwired: 2 in, 2 out]
            n3459 = local read "bs"() -> (w4434:string)
            n3460 = local read "as"() -> (w4433:string)
            n3461 = property on="CH-POWER +" class="DigNum (strict)"("Caption.Text"=w4413) -> ()  [unwired: 2 in, 2 out]
            n3462 = property on="CH-POWER -" class="DigNum (strict)"("Caption.Text"=w4412) -> ()  [unwired: 2 in, 2 out]
            n3463 = property on="CH-HEATER" class="DigNum (strict)"("Caption.Text"=w4411) -> ()  [unwired: 2 in, 2 out]
            n3464 = property on="CH-HUMIDITY DRY" class="DigNum (strict)"("Caption.Text"=w4410) -> ()  [unwired: 2 in, 2 out]
            n3465 = property on="CH-HUMIDITY WET" class="DigNum (strict)"("Caption.Text"=w4409) -> ()  [unwired: 2 in, 2 out]
            n3466 = local read "S 60"() -> (w4445:string)
            n3467 = local read "S 54"() -> (w4455:string)
            n3468 = Concatenate Strings(w4434, "\r", w4433) -> ()  [unwired: 1 out]
            n3469 = Concatenate Strings(w4455, w4445) -> ()  [unwired: 1 out]
            n3470 = local read "S 77"() -> (→"String 43":string)
            n3471 = local read "S 76"() -> (w4428:string)
            n3472 = local read "S 78"() -> (w4427:string)
            n3473 = local read "S 71"() -> (w4439:string)
            n3474 = local read "S 66"() -> (w4444:string)
            n3475 = local read "S 67"() -> (w4443:string)
            n3476 = local read "S 68"() -> (w4442:string)
            n3477 = local read "S 69"() -> (w4441:string)
            n3478 = local read "S 70"() -> (w4440:string)
            n3479 = property on="AIR TEMP" class="DigNum (strict)"("Caption.Text"=w4427) -> ()  [unwired: 2 in, 2 out]
            n3480 = property on="Set Strk" class="DigNum (strict)"("Caption.Text"=w4428) -> ()  [unwired: 2 in, 2 out]
            n3481 = property on="FRIC. FORCE :" class="DigNum (strict)"("Caption.Text"=w4444) -> ()  [unwired: 2 in, 2 out]
            n3482 = property on="TEMPERATURE :" class="DigNum (strict)"("Caption.Text"=w4443) -> ()  [unwired: 2 in, 2 out]
            n3483 = property on="SPEED OUT:" class="DigNum (strict)"("Caption.Text"=w4442) -> ()  [unwired: 2 in, 2 out]
            n3484 = property on="AIR TEMPERATURE :" class="DigNum (strict)"("Caption.Text"=w4441) -> ()  [unwired: 2 in, 2 out]
            n3485 = property on="HUMIDITY:" class="DigNum (strict)"("Caption.Text"=w4440) -> ()  [unwired: 2 in, 2 out]
            n3486 = property on="EDIT" class="Bool (strict)"("Boolean Text.Text"=w4439) -> ()  [unwired: 2 in, 2 out]
            n3487 = local read "S 79"() -> (w4426:string)
          }
          frame #2 {
          }
        }
        n3488 = local write "Lan flag"(10.0 ("Lan flag")) -> ()
      }
      frame Enabled {
      }
    }
    n3489 = Wait (ms)(milliseconds to wait=u32 2000) -> ()  [unwired: 1 out]
    n3490 = local read "Quit"() -> (w4229:bool)
  }
  n3491 = disable-structure shown="Disabled" {
    frame Disabled {
      n3492 = while {
        tunnel: [w4457] -> _
        i -> [w4457]
        stop <- w4456 continue-if-true
        n3493 = Wait (ms)(milliseconds to wait=u32 50) -> ()  [unwired: 1 out]
        n3494 = stacked-sequence {
          frame #0 {
            # "Controls Text color"
            # "Controls BG color"
            n3495 = property on="FILE" class="Str"("Text.Text Colors:Text Color"="SC  Text") -> ()  [unwired: 2 in, 2 out]
            n3496 = property on="Fuel Discription :" class="Str"("Text.Text Colors:Text Color"="SC  Text") -> ()  [unwired: 2 in, 2 out]
            n3497 = property on="tested by" class="Str"("Text.Text Colors:Text Color"="SC  Text") -> ()  [unwired: 2 in, 2 out]
            n3498 = property on="Remarks :" class="Str"("Text.Text Colors:Text Color"="SC  Text") -> ()  [unwired: 2 in, 2 out]
            n3499 = property class="DigNum (strict)"("Numeric Text.Text Colors:BG Color"="NC BG") -> ()  [unwired: 2 in, 2 out]
            n3500 = property class="DigNum (strict)"("Numeric Text.Text Colors:BG Color"="NC BG") -> ()  [unwired: 2 in, 2 out]
            n3501 = property class="DigNum (strict)"("Numeric Text.Text Colors:BG Color"="NC BG") -> ()  [unwired: 2 in, 2 out]
            n3502 = property class="DigNum (strict)"("Numeric Text.Text Colors:BG Color"="NC BG") -> ()  [unwired: 2 in, 2 out]
            n3503 = property class="DigNum (strict)"("Numeric Text.Text Colors:BG Color"="NC BG") -> ()  [unwired: 2 in, 2 out]
            n3504 = property class="DigNum (strict)"("Numeric Text.Text Colors:BG Color"="NC BG") -> ()  [unwired: 2 in, 2 out]
            n3505 = property class="DigNum (strict)"("Numeric Text.Text Colors:BG Color"="NC BG") -> ()  [unwired: 2 in, 2 out]
            n3506 = property class="DigNum (strict)"("Numeric Text.Text Colors:BG Color"="NC BG") -> ()  [unwired: 2 in, 2 out]
            n3507 = property class="DigNum (strict)"("Numeric Text.Text Colors:BG Color"="NC BG") -> ()  [unwired: 2 in, 2 out]
            n3508 = property class="DigNum (strict)"("Numeric Text.Text Colors:BG Color"="NC BG") -> ()  [unwired: 2 in, 2 out]
            n3509 = property class="DigNum (strict)"("Numeric Text.Text Colors:BG Color"="NC BG") -> ()  [unwired: 2 in, 2 out]
            n3510 = property class="DigNum (strict)"("Numeric Text.Text Colors:BG Color"="NC BG") -> ()  [unwired: 2 in, 2 out]
            n3511 = property on="FILE" class="Str"("Text.Text Colors:BG Color"="SC BG 3") -> ()  [unwired: 2 in, 2 out]
            n3512 = property on="Fuel Discription :" class="Str"("Text.Text Colors:BG Color"="SC BG 3") -> ()  [unwired: 2 in, 2 out]
            n3513 = property on="tested by" class="Str"("Text.Text Colors:BG Color"="SC BG 3") -> ()  [unwired: 2 in, 2 out]
            n3514 = property on="Remarks :" class="Str"("Text.Text Colors:BG Color"="SC BG 3") -> ()  [unwired: 2 in, 2 out]
            n3515 = property class="DigNum (strict)"("Numeric Text.Text Colors:Text Color"="NC Text") -> ()  [unwired: 2 in, 2 out]
            n3516 = property class="DigNum (strict)"("Numeric Text.Text Colors:Text Color"="NC Text") -> ()  [unwired: 2 in, 2 out]
            n3517 = property class="DigNum (strict)"("Numeric Text.Text Colors:Text Color"="NC Text") -> ()  [unwired: 2 in, 2 out]
            n3518 = property class="DigNum (strict)"("Numeric Text.Text Colors:Text Color"="NC Text") -> ()  [unwired: 2 in, 2 out]
            n3519 = property class="DigNum (strict)"("Numeric Text.Text Colors:Text Color"="NC Text") -> ()  [unwired: 2 in, 2 out]
            n3520 = property class="DigNum (strict)"("Numeric Text.Text Colors:Text Color"="NC Text") -> ()  [unwired: 2 in, 2 out]
            n3521 = property class="DigNum (strict)"("Numeric Text.Text Colors:Text Color"="NC Text") -> ()  [unwired: 2 in, 2 out]
            n3522 = property class="DigNum (strict)"("Numeric Text.Text Colors:Text Color"="NC Text") -> ()  [unwired: 2 in, 2 out]
            n3523 = property class="DigNum (strict)"("Numeric Text.Text Colors:Text Color"="NC Text") -> ()  [unwired: 2 in, 2 out]
            n3524 = property class="DigNum (strict)"("Numeric Text.Text Colors:Text Color"="NC Text") -> ()  [unwired: 2 in, 2 out]
            n3525 = property class="DigNum (strict)"("Numeric Text.Text Colors:Text Color"="NC Text") -> ()  [unwired: 2 in, 2 out]
            n3526 = property class="DigNum (strict)"("Numeric Text.Text Colors:Text Color"="NC Text") -> ()  [unwired: 2 in, 2 out]
            n3527 = property class="DigNum (strict)"("Numeric Text.Text Colors:Text Color"="NI Text  2") -> ()  [unwired: 2 in, 2 out]
            n3528 = property class="DigNum (strict)"("Numeric Text.Text Colors:Text Color"="NI Text  2") -> ()  [unwired: 2 in, 2 out]
            n3529 = property class="DigNum (strict)"("Numeric Text.Text Colors:Text Color"="NI Text  2") -> ()  [unwired: 2 in, 2 out]
            n3530 = property class="DigNum (strict)"("Numeric Text.Text Colors:Text Color"="NI Text  2") -> ()  [unwired: 2 in, 2 out]
            n3531 = property class="DigNum (strict)"("Numeric Text.Text Colors:Text Color"="NI Text  2") -> ()  [unwired: 2 in, 2 out]
            n3532 = property class="DigNum (strict)"("Numeric Text.Text Colors:Text Color"="NI Text  2") -> ()  [unwired: 2 in, 2 out]
            n3533 = property class="DigNum (strict)"("Numeric Text.Text Colors:Text Color"="NI Text  2") -> ()  [unwired: 2 in, 2 out]
            n3534 = property class="DigNum (strict)"("Numeric Text.Text Colors:Text Color"="NI Text  2") -> ()  [unwired: 2 in, 2 out]
            n3535 = property class="DigNum (strict)"("Numeric Text.Text Colors:Text Color"="NI Text  2") -> ()  [unwired: 2 in, 2 out]
            n3536 = property class="DigNum (strict)"("Numeric Text.Text Colors:Text Color"="NI Text  2") -> ()  [unwired: 2 in, 2 out]
            n3537 = property class="DigNum (strict)"("Numeric Text.Text Colors:Text Color"="NI Text  2") -> ()  [unwired: 2 in, 2 out]
            n3538 = property class="DigNum (strict)"("Numeric Text.Text Colors:Text Color"="NI Text  2") -> ()  [unwired: 2 in, 2 out]
